vi "ZMC Get Axis States.vi"(8 "error in (no error)":errorcluster caption="错误输入（无错误）", 9 "pstrstates":T1, 10 "iaxis":u8, 11 "handle":u32) -> (0 "error out":errorcluster caption="错误输出", 1 "pstrstates out":T1, 2 "function return":i32, 3 "handle out":u32)   [LabVIEW 2019, in "zauxdll.lvlib"]
doc: "int32 __stdcall ZMC_GetAxisStates(ZMC_HANDLE handle, uint8 iaxis, struct_AxisStates* pstrstates);"
uses:
  zauxdll.lvlib
  zmotion.dll
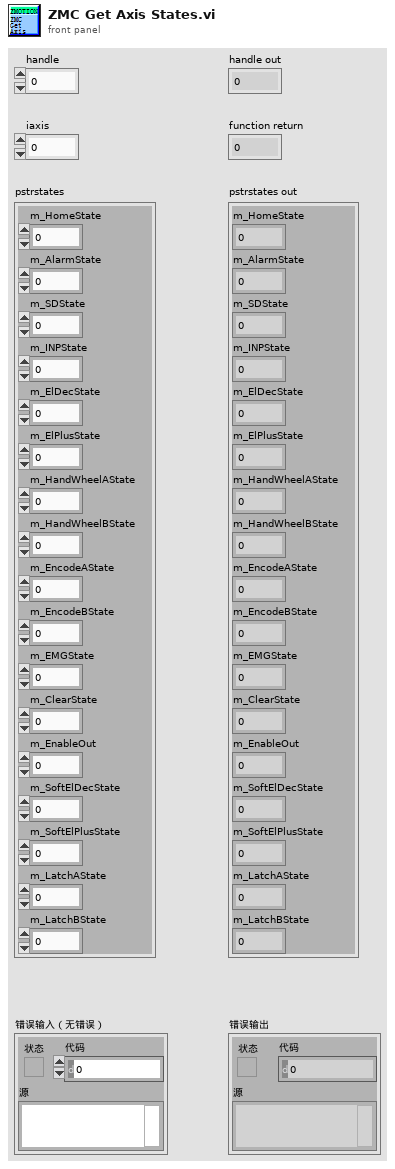
[diagram p1: front panel]
types:
  T1 = cluster{"m_HomeState":u8, "m_AlarmState":u8, "m_SDState":u8, "m_INPState":u8, "m_ElDecState":u8, "m_ElPlusState":u8, "m_HandWheelAState":u8, "m_HandWheelBState":u8, "m_EncodeAState":u8, "m_EncodeBState":u8, "m_EMGState":u8, "m_ClearState":u8, "m_EnableOut":u8, "m_SoftElDecState":u8, "m_SoftElPlusState":u8, "m_LatchAState":u8, "m_LatchBState":u8}
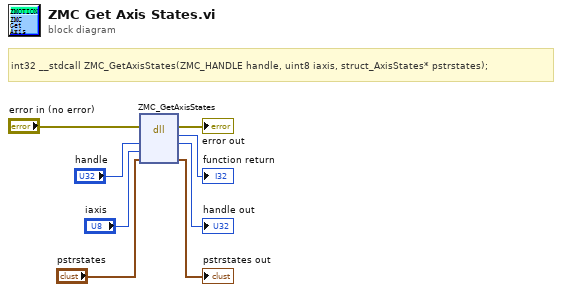
[diagram p0: block diagram]
diagram:
  # "int32 __stdcall ZMC_GetAxisStates(ZMC_HANDLE handle, uint8 iaxis, struct_AxisStates* pstrstates);"
  n1 = dll-call lib="C:/Users/VIC/Desktop/Standar Program/System/LLB/zmotion/zaux/zmotion.*" fn="ZMC_GetAxisStates"(error in="error in (no error)", "handle"="handle", "iaxis"="iaxis", "pstrstates"="pstrstates") -> (error out=→"error out":errorcluster, →"function return":i32, "handle"=→"handle out":u32, "pstrstates"=→"pstrstates out":T1)  [unwired: 3 in, 1 out]
